vi "TDS Waveform Output Write.vi"(6 "Waveform Settings":T1={"Frequency"=0.0, "Amplitude"=0.0, "DC Offset"=0.0, "Duty Cycle"=-1.0, "Number of Samples"=-1, "Sample Rate"=-1}, 8 "error in (no error)":errorcluster, 9 "Waveform Type":string(combo), 10 "Signal InstConfig":string, 11 "Address":string) -> (0 "error out":errorcluster)   [LabVIEW 2025, in "Interface Functions.lvlib"]
uses:
  Interface Functions.lvlib
  <vilib>/Utility/error.llb/Trim Whitespace One-Sided.vi
panel:
  # "Waveform Output Write"
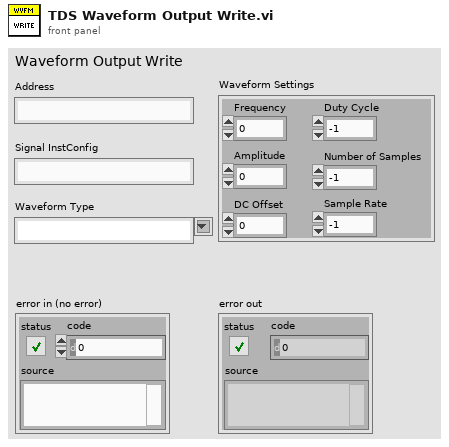
[diagram p1: front panel]
types:
  T1 = cluster{"Frequency":dbl, "Amplitude":dbl, "DC Offset":dbl, "Duty Cycle":dbl, "Number of Samples":i32, "Sample Rate":i32}
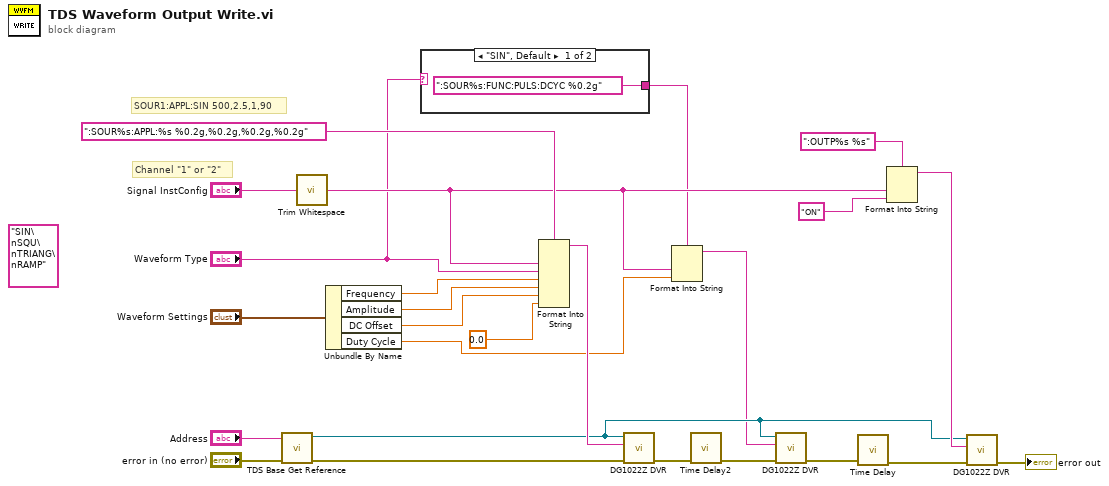
[diagram p0: block diagram]
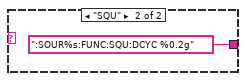
[diagram p2: hidden frame]
diagram:
  (unwired) "SIN\nSQU\nTRIANG\nRAMP" ("multi-line string")
  # "SOUR1:APPL:SIN 500,2.5,1,90"
  # "Channel \"1\" or \"2\""
  n1 = call "TDS Base Get Reference.vi"("error in (no error)"="error in (no error)", "Address"="Address") -> ("error out"=w22:errorcluster, "Reference"=w9:refnum<visa-resource-name>)  [unwired: 8 in]
  n2 = call <vilib>:"Trim Whitespace.vi"("string"="Signal InstConfig") -> ("trimmed string"=w8:string)  [unwired: 1 in]
  n3 = Unbundle By Name("Waveform Settings") -> ("Frequency"=w20:dbl, "Amplitude"=w19:dbl, "DC Offset"=w18:dbl, "Duty Cycle"=w5:dbl)
  n4 = case shown="\"SIN\", Default" "Waveform Type" {
    tunnel: [":SOUR%s:FUNC:PULS:DCYC %0.2g" ("format string") ":SOUR%s:FUNC:SQU:DCYC %0.2g" ("format string")] -> w6
    frame "SIN", Default {
    }
    frame "SQU" {
    }
  }
  n5 = Format Into String(format string=":SOUR%s:APPL:%s %0.2g,%0.2g,%0.2g,%0.2g", w8, "Waveform Type", w20, w19, w18, 0.0 ("Duty Cycle")) -> (resulting string=w17:string)  [unwired: 2 in, 1 out]
  n6 = call "DG1022Z DVR.vi"("error in (no error)"=w22, "write buffer"=w17, "VISA resource name"=w9) -> ("error out"=w3:errorcluster)  [unwired: 7 in, 1 out]
  n7 = Format Into String(format string=w6, w8, w5) -> (resulting string=w4:string)  [unwired: 2 in, 1 out]
  n8 = call "Time Delay2"("error in (no error)"=w3) -> ("error out"=w2:errorcluster)  [unwired: 10 in]
  n9 = call "DG1022Z DVR.vi"("error in (no error)"=w2, "write buffer"=w4, "VISA resource name"=w9) -> ("error out"=w1:errorcluster)  [unwired: 7 in, 1 out]
  n10 = call "Time Delay"("error in (no error)"=w1) -> ("error out"=w12:errorcluster)  [unwired: 10 in]
  n11 = Format Into String(format string=":OUTP%s %s", w8, "ON") -> (resulting string=w13:string)  [unwired: 2 in, 1 out]
  n12 = call "DG1022Z DVR.vi"("error in (no error)"=w12, "write buffer"=w13, "VISA resource name"=w9) -> ("error out"=→"error out":errorcluster)  [unwired: 7 in, 1 out]
